vi "Write LED state.vi"(8 "error in (no error)":errorcluster, 9 "state":bool, 10 "LED":u16(ring)=1 items=["D1 (LED1)"=1, "D2 (LED2)"=2], 11 "connection ID":i32=-1) -> (0 "error out":errorcluster, 3 "link_fd out":i32)   [LabVIEW 2009, in "MicroDAQ.lvlib"]
doc: "This function sets states of MicroDAQ built in D1 and D2 LEDs."
uses:
  <instrlib>/MicroDAQ/MicroDAQ.lvlib
  <instrlib>/MicroDAQ/Mlink library wraper/mlink.lvlib
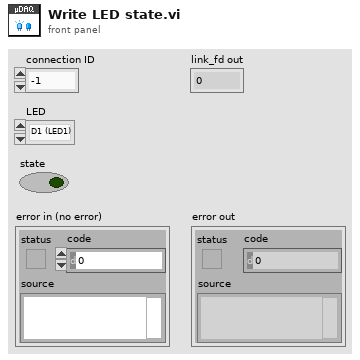
[diagram p1: front panel]
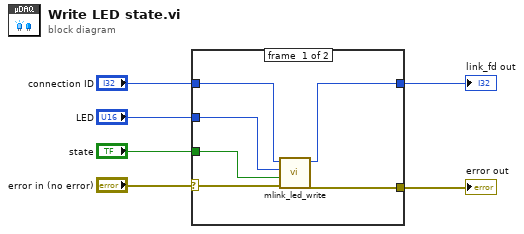
[diagram p0: block diagram]
diagram:
  n1 = case shown="No Error" "error in (no error)" {
    selector: "error in (no error)" -> [w12 w13]
    tunnel: "state" -> [w11 _]
    tunnel: "LED" -> [w10 _]
    tunnel: "connection ID" -> [w9 w14]
    tunnel: [w8 w13] -> w2
    tunnel: [w7 w14] -> w1
    frame #0 {
      n2 = call <instrlib>:"mlink_led_write.vi"("error in (no error)"=w12, "state"=w11, "LED"=w10, "connection ID"=w9) -> ("error out"=w8:errorcluster, "link_fd out"=w7:i32)  [unwired: 6 in]
    }
    frame #1 {
    }
  }
  "error out" <- w2
  "link_fd out" <- w1
